vi "Module Type.vi"(11 "GenericGuiAO in":refnum<class "GenericGuiDO.lvclass">) -> (2 "Module Type":string)   [LabVIEW 2020, in "VolatusDAQGenericGUI.lvlib" / "GenericGuiDO.lvclass"]
uses:
  GenericGuiDO.lvclass
  GenericGuiDO.lvclass/GenericGuiDO.ctl
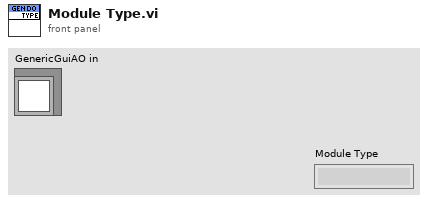
[diagram p1: front panel]
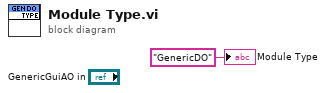
[diagram p0: block diagram]
diagram:
  "Module Type" <- "GenericDO" ("Module Type")
